vi "Write Element of Intervals.vi"(8 "error in (no error)":errorcluster, 9 "Interval":T2, 10 "Parameters":T1, 11 "Cron in":refnum<class "Cron.lvclass">) -> (0 "error out":errorcluster, 3 "Cron out":refnum<class "Cron.lvclass">)   [LabVIEW 2013, in "openCron.lvlib" / "Cron.lvclass"]
uses:
  Cron.lvclass
  Cron Interval -- enum.ctl
  Cron Interval -- cluster.ctl
  Cron.lvclass/Cron.ctl
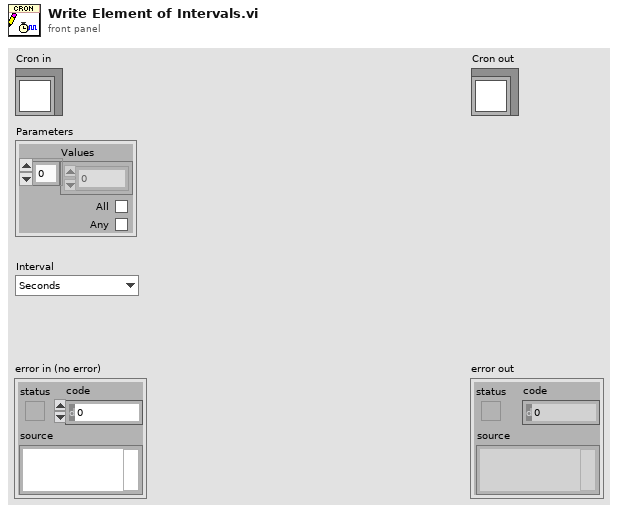
[diagram p1: front panel]
types:
  T1 = typedef "openCron.lvlib/Cron.lvclass/Cron Interval -- cluster.ctl" = cluster{"Values":i32[], "All":bool, "Any":bool}
  T2 = typedef "openCron.lvlib/Cron.lvclass/Cron Interval -- enum.ctl" = enum16{"Seconds", "Minutes", "Hours", "Day of Month", "Month", "Day of Week", "Year"}
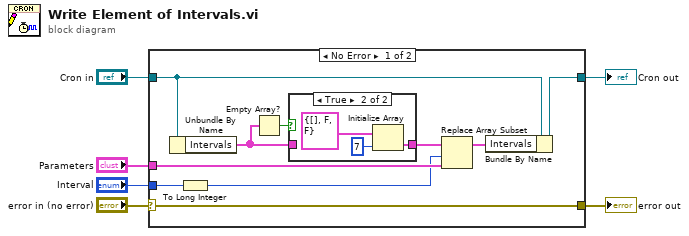
[diagram p0: block diagram]
diagram:
  n1 = case shown="No Error" "error in (no error)" {
    selector: "error in (no error)" -> [w16 w21]
    tunnel: [w16 w21] -> w5
    tunnel: [w12 w22] -> w3
    tunnel: "Cron in" -> [w15 w22]
    tunnel: "Parameters" -> [w13 _]
    tunnel: "Interval" -> [w8 _]
    frame No Error {
      n2 = Unbundle By Name(w15) -> ("Intervals"=w9:T1[])
      n3 = To Long Integer(number=w8) -> (32bit integer=w7:i32)
      n4 = Empty Array?(array=w9) -> (empty?=w11:bool)
      n5 = case shown="True" w11 {
        tunnel: [w17 w18] -> w10
        tunnel: w9 -> [w17 _]
        frame False {
        }
        frame True {
          n6 = Initialize Array(T1 {"Values"=[], "All"=FALSE, "Any"=FALSE} ("Interval"), 7 ("dimension size")) -> (w18:T1[])
        }
      }
      n7 = Replace Array Subset(array=w10, new element=w13, index=w7) -> (w14:T1[])
      n8 = Bundle By Name(cluster=w15, "Intervals"=w14) -> (w12:refnum<class "Cron.lvclass">)
    }
    frame Error {
    }
  }
  "error out" <- w5
  "Cron out" <- w3
